vi "Update document.vi"(8 "error in (no error)":errorcluster caption="entrée d'erreur (pas d'erreur)", 11 "Firebase (Default) en entrée":refnum<class "Firebase Driver.lvclass">) -> (0 "error out":errorcluster caption="sortie d'erreur", 3 "Firebase (Default) en sortie":refnum<class "Firebase Driver.lvclass">)   [LabVIEW 2020, in "Library Instrument & Equipement.lvlib" / "Library FireBase.lvlib" / "Firebase Driver.lvclass"]
uses:
  Firebase Driver.lvclass
  Firebase Driver.lvclass/Firebase Driver.ctl
  JSON API/JSON Value/Set from JSON string.vi
  JSON API/Variant JSON/Variant to JSON.vi
  JSON API/JSON Value/Get Item by name array.vi
  JSON API/JSON Value/JSON Value.lvclass
  JSON API/Get Polymorphic/JSON GetSet.lvlib
  JSON API/Variant JSON/Variant JSON.lvlib
  Http Altyor/Session.lvclass
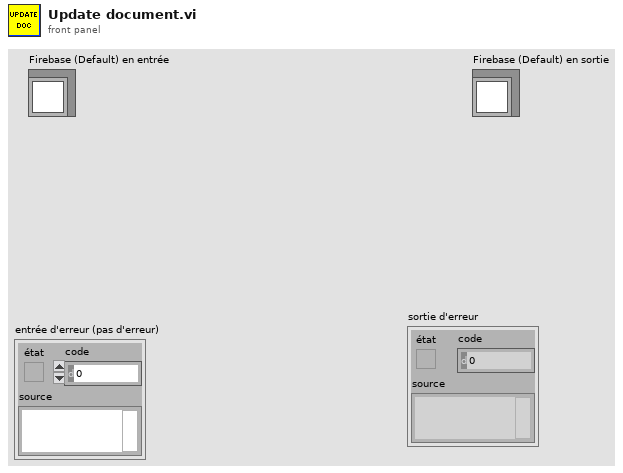
[diagram p1: front panel]
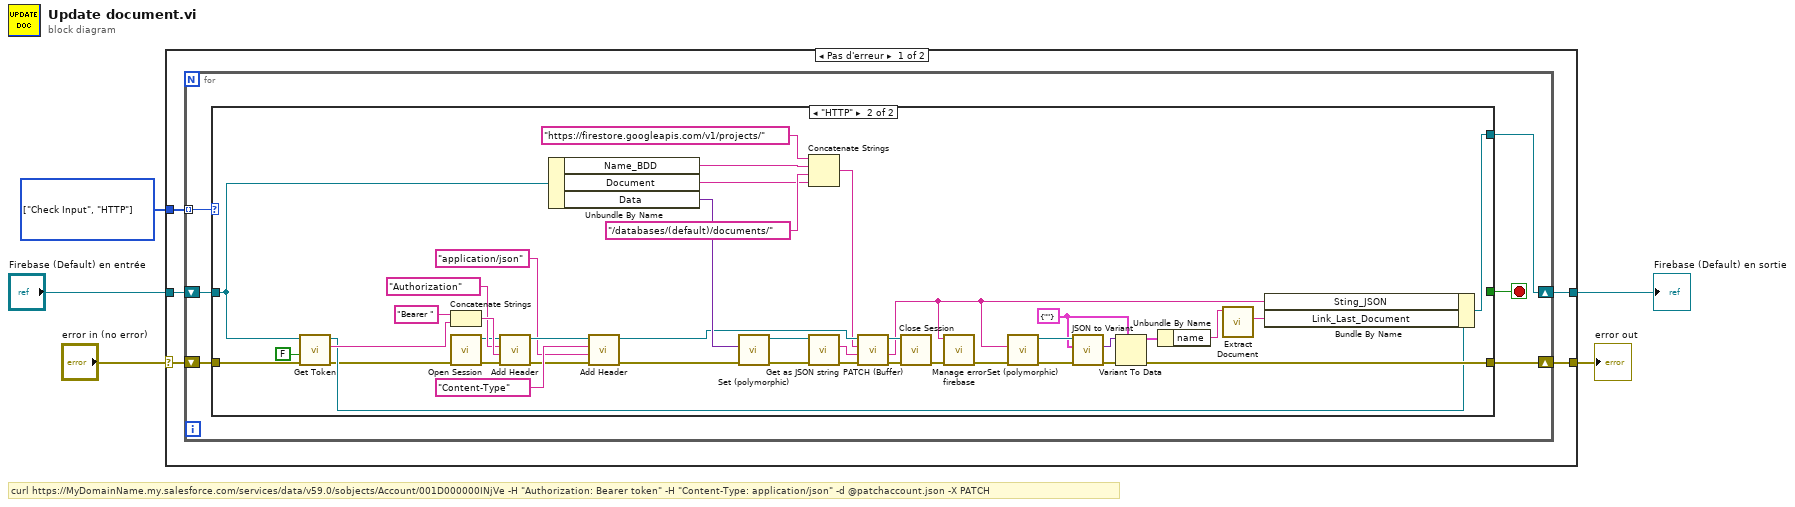
[diagram p0: block diagram]
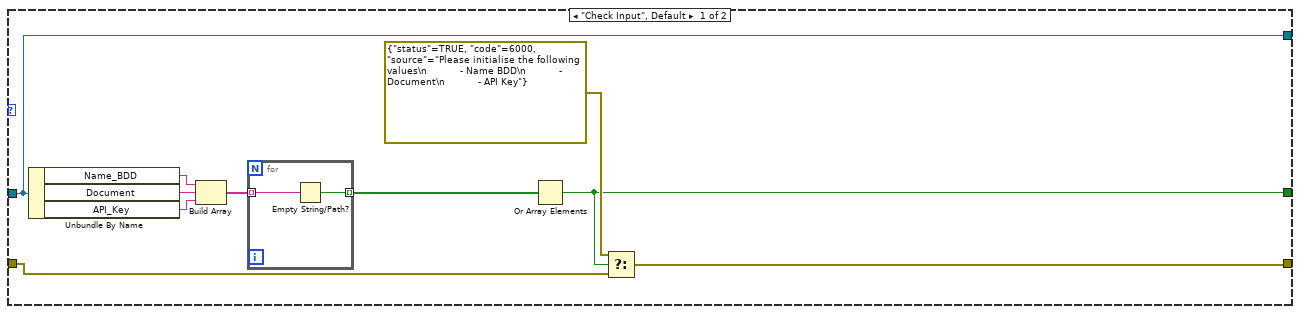
[diagram p2: hidden frame]
diagram:
  w1 = enum16{"Check Input", "HTTP"}[] [enum."Check Input", enum."HTTP"] items=["Check Input", "HTTP"]
  # "curl https://MyDomainName.my.salesforce.com/services/data/v59.0/sobjects/Account/001D000000INjVe -H \"Authorization: Bearer token\" -H \"Content-Type: application/json\" -d @patchaccount.json -X PATCH"
  n1 = case shown="Pas d'erreur" "error in (no error)" {
    selector: "error in (no error)" -> [w10 w72]
    tunnel: [w9 w72] -> w4
    tunnel: "Firebase (Default) en entrée" -> [w8 w71]
    tunnel: [w7 w71] -> w2
    tunnel: w1 -> [w6 _]
    frame No Error {
      n2 = for {
        shift-right: [w13] -> w9
        shift-left: w10 -> [w16]
        shift-right: [w14] -> w7
        shift-left: w8 -> [w15]
        tunnel: w6 -> [w12] mode=indexing
        stop <- w11 stop-if-true
        n3 = case shown="\"HTTP\"" w12 {
          tunnel: w16 -> [w22 w67]
          tunnel: w15 -> [w20 w51]
          tunnel: [w20 w64] -> w14
          tunnel: [w21 w55] -> w13
          tunnel: [w23 _] -> w11
          frame "Check Input", Default {
            n4 = Unbundle By Name(w20) -> ("Name_BDD"=w19:string, "Document"=w18:string, "API_Key"=w17:string)
            n5 = Build Array(w19, w18, w17) -> (w26:string[])
            n6 = for {
              tunnel: w26 -> [w27] mode=indexing
              tunnel: [w28] -> w25 mode=indexing
              n7 = Empty String/Path?(string/path=w27) -> (empty?=w28:bool)
            }
            n8 = Or Array Elements(Boolean array=w25) -> (logical OR=w23:bool)
            n9 = Select(t=errorcluster {"status"=TRUE, "code"=6000, "source"="Please initialise the following values\n           - Name BDD\n           - Document\n           - API Key"} ("cas vrai"), s=w23, f=w22) -> (s? t:f=w21:errorcluster)
          }
          frame "HTTP" {
            w59 = cluster{"name":string} {"name"=""}
            n10 = call-dynamic "Get Token.vi"("error in (no error)"=w67, "Reset"=FALSE, "Build Library FireBase.lvlib:Firebase (Default) IN"=w51) -> ("error out"=w47:errorcluster, "idToken"=w52:string, "Build Library FireBase.lvlib:Firebase (Default) Out"=w50:refnum<class "Firebase Driver.lvclass">)  [unwired: 6 in]
            n11 = Concatenate Strings("Bearer " ("chaîne"), w52) -> (w46:string)
            n12 = call "Open Session.vi"("error in"=w47) -> ("error out"=w30:errorcluster, "session"=w44:refnum<class "Session.lvclass">)  [unwired: 9 in]
            n13 = call "Add Header.vi"("error in"=w30, "value"=w46, "header"="Authorization", "session in"=w44) -> ("error out"=w40:errorcluster, "session out"=w43:refnum<class "Session.lvclass">)  [unwired: 6 in]
            n14 = Unbundle By Name(w51) -> ("Name_BDD"=w68:string, "Document"=w49:string, "Data"=w65:variant)
            n15 = call "Add Header.vi"("error in"=w40, "value"="application/json", "header"="Content-Type", "session in"=w43) -> ("error out"=w39:errorcluster, "session out"=w35:refnum<class "Session.lvclass">)  [unwired: 6 in]
            n16 = call-poly "Set (polymorphic).vi"("error in (no error)"=w39, "Variant"=w65) -> ("error out"=w53:errorcluster, "JSON Value out"=w54:refnum<class "JSON Value.lvclass">)  [unwired: 8 in]
            n17 = Concatenate Strings("https://firestore.googleapis.com/v1/projects/" ("string"), w68, "/databases/(default)/documents/" ("string"), w49) -> (w34:string)
            n18 = call "Get as JSON string.vi"("error in (no error)"=w53, "JSON Value in"=w54) -> ("error out"=w36:errorcluster, "<JSON>"=w33:string)  [unwired: 8 in]
            n19 = call "PATCH (Buffer).vi"("error in"=w36, "buffer"=w33, "url"=w34, "Session In"=w35) -> ("error out"=w37:errorcluster, "body"=w31:string, "Session Out"=w32:refnum<class "Session.lvclass">)  [unwired: 3 in, 2 out]
            n20 = call "Close Session.vi"("error in"=w37, "Session In"=w32) -> ("error out"=w38:errorcluster)  [unwired: 9 in]
            n21 = call "Manage error firebase.vi"("error in (no error)"=w38, "Body"=w31) -> ("error out"=w56:errorcluster)  [unwired: 9 in]
            n22 = call-poly "Set (polymorphic).vi"("error in (no error)"=w56, "JSON stream"=w31) -> ("error out"=w60:errorcluster, "JSON Value out"=w63:refnum<class "JSON Value.lvclass">)  [unwired: 7 in, 1 out]
            n23 = call "JSON to Variant.vi"("error in (no error)"=w60, "Variant (Data Type)"=w59, "JSON Value"=w63) -> ("error out"=w61:errorcluster, "Variant out"=w62:variant)  [unwired: 7 in]
            n24 = Variant To Data(error in=w61, type=w59, Variant=w62) -> (data=w58:cluster{"name":string}, error out=w55:errorcluster)
            n25 = Unbundle By Name(w58) -> ("name"=w57:string)
            n26 = call "Extract Document.vi"("Name"=w57) -> ("Source"=w48:string)  [unwired: 9 in, 1 out]
            n27 = Bundle By Name(cluster=w50, "Sting_JSON"=w31, "Link_Last_Document"=w48) -> (w64:refnum<class "Firebase Driver.lvclass">)
          }
        }
      }
    }
    frame Error {
    }
  }
  "error out" <- w4
  "Firebase (Default) en sortie" <- w2
